vi "Chart[Template].Export.vi"(8 "error in (no error)":errorcluster, 10 "Export Folder Path":path, 11 "DisplayWaveforms":refnum<class "DisplayWaveforms.lvclass">) -> (0 "error out":errorcluster, 3 "DisplayWaveforms out":refnum<class "DisplayWaveforms.lvclass">)   [LabVIEW 2020, in "DisplayWaveform.lvlib" / "DisplayWaveforms.lvclass"]
doc: "Export Chart Data"
uses:
  DisplayWaveforms.lvclass
  DisplayWaveforms.lvclass/DisplayWaveforms.ctl
  <vilib>/Utility/file.llb/Write Delimited Spreadsheet (DBL).vi
panel:
  in  "Pause Charts":bool
  # "For instructions on how to use the JKI State Machine Objects, examples and video tutorials, visit:\nhttp://jki.net/state-machine-objects/\n\nJKI State Machine Objects™\nhttp://jki.net/state-machine-objects/\nCopyright (C) 2005-2015, JKI <info@jki.net>\nALL RIGHTS RESERVED"
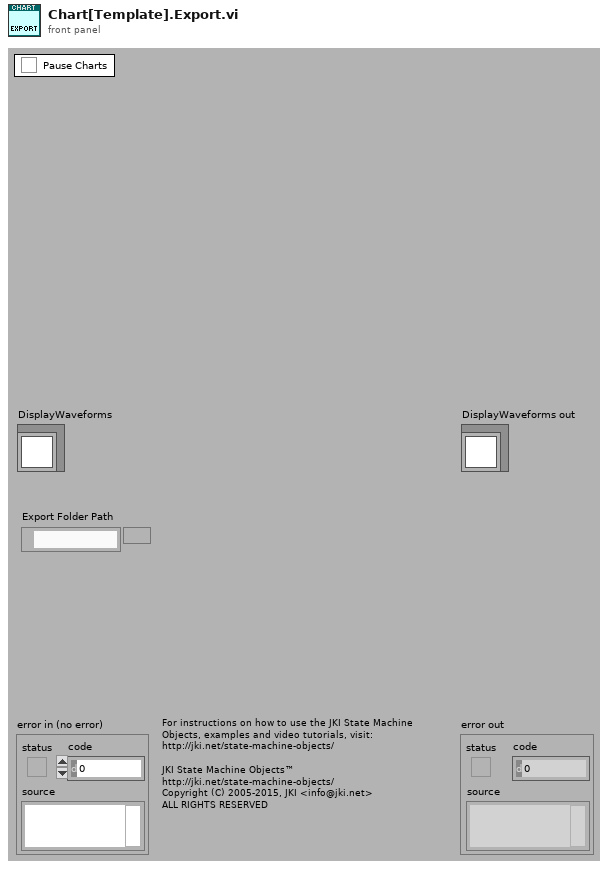
[diagram p1: front panel]
types:
  T1 = typedef "DisplayWaveform.lvlib/DisplayWaveforms.lvclass/PublicEvents--Cluster.ctl" = cluster{"Chart Cleared":refnum<user-event>, "Chart Exported":refnum<user-event>, "ChartParams Set":refnum<user-event>}
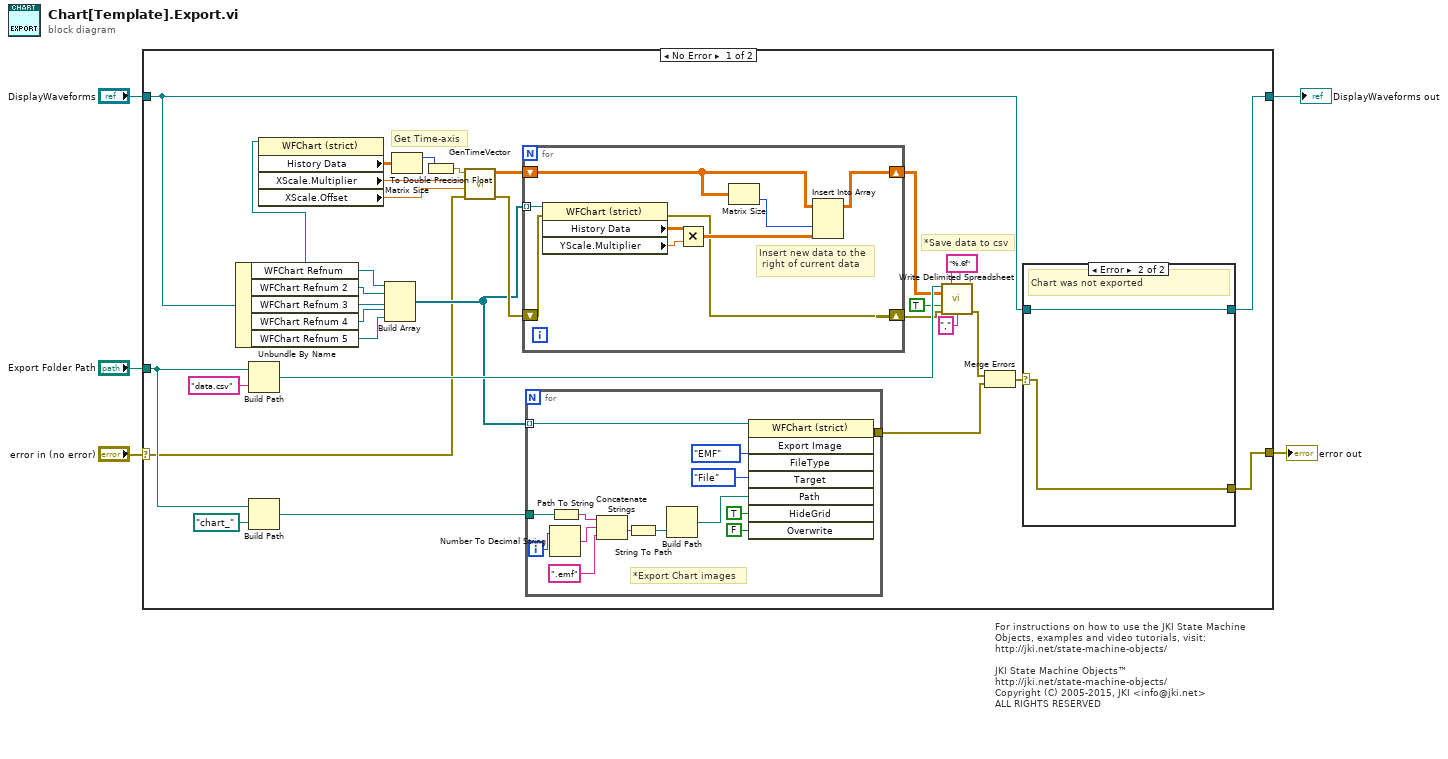
[diagram p0: block diagram]
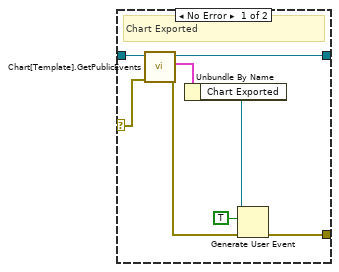
[diagram p2: hidden frame]
diagram:
  # "For instructions on how to use the JKI State Machine Objects, examples and video tutorials, visit:\nhttp://jki.net/state-machine-objects/\n\nJKI State Machine Objects™\nhttp://jki.net/state-machine-objects/\nCopyright (C) 2005-2015, JKI <info@jki.net>\nALL RIGHTS RESERVED"
  n1 = case shown="No Error" "error in (no error)" {
    selector: "error in (no error)" -> [w8 w69]
    tunnel: "DisplayWaveforms" -> [w27 w70]
    tunnel: [w35 w69] -> w4
    tunnel: [w34 w70] -> w3
    tunnel: "Export Folder Path" -> [w25 _]
    frame No Error {
      # "Get Time-axis"
      # "*Save data to csv"
      n2 = Unbundle By Name(w27) -> ("WFChart Refnum"=w24:refnum<vi>, "WFChart Refnum 2"=w23:refnum<vi>, "WFChart Refnum 3"=w22:refnum<vi>, "WFChart Refnum 4"=w21:refnum<vi>, "WFChart Refnum 5"=w20:refnum<vi>)
      n3 = Build Path(base path=w25, name or relative path="data.csv" ("string")) -> (appended path=w31:path)
      n4 = Build Path(base path=w25, name or relative path=path "chart_") -> (appended path=w17:path)
      n5 = property on="Property Node" class="WFChart (strict)"(reference=w24) -> ("History Data"=w32:dbl[][], "XScale.Multiplier"=w16:dbl, "XScale.Offset"=w15:dbl)  [unwired: 1 in, 2 out]
      n6 = Build Array(w24, w23, w22, w21, w20) -> (w9:refnum<vi>[])
      n7 = Matrix Size(0:w32) -> (1:w6:i32)  [unwired: 1 out]
      n8 = To Double Precision Float(number=w6) -> (double precision float=w14:dbl)
      n9 = call "GenTimeVector.vi"("error in (no error)"=w8, "Offset"=w15, "Multiplier - dT"=w16, "# of elements"=w14) -> ("error out"=w12:errorcluster, "Time Vector"=w13:dbl[][])  [unwired: 6 in]
      n10 = for {
        shift-right: [w39] -> w11
        shift-left: w13 -> [w42]
        shift-right: [w37] -> w10
        shift-left: w12 -> [w38]
        tunnel: w9 -> [w36] mode=indexing
        # "Insert new data to the\n right of current data"
        n11 = property on="Property Node" class="WFChart (strict)"(reference=w36, error in=w38) -> (error out=w37:errorcluster, "History Data"=w44:dbl[][], "YScale.Multiplier"=w43:dbl)  [unwired: 1 out]
        n12 = Multiply(x=w44, y=w43) -> (x*y=w40:dbl[][])
        n13 = Matrix Size(0:w42) -> (2:w41:i32)  [unwired: 1 out]
        n14 = Insert Into Array(array=w42, index (col)=w41, new element=w40) -> (w39:dbl[][])  [unwired: 1 in]
      }
      n15 = for {
        tunnel: w9 -> [w55] mode=indexing
        tunnel: [w54] -> w19
        tunnel: w17 -> [w46]
        i -> [w50]
        # "*Export Chart images"
        n16 = Number To Decimal String(number=w50) -> (decimal integer string=w49:string)  [unwired: 1 in]
        n17 = Path To String(path=w46) -> (string=w45:string)
        n18 = Concatenate Strings(w45, w49, ".emf" ("string")) -> (w51:string)
        n19 = String To Path(string=w51) -> (path=w52:path)
        n20 = Build Path(name or relative path=w52) -> (appended path=w47:path)  [unwired: 1 in]
        n21 = invoke on="Invoke Node" class="WFChart (strict)" method="Export Image"(reference=w55, "FileType"=enum32{"BMP", "EPS", "EMF", "PICT"}."EMF" ("File Type"), "Target"=enum32{"File", "Clipboard"}."File", "Path"=w47, "HideGrid"=TRUE ("Hide Grid"), "Overwrite"=FALSE ("Always Overwrite")) -> (error out=w54:errorcluster)  [unwired: 2 in, 7 out]
      }
      n22 = call-poly <vilib>:"Write Delimited Spreadsheet.vi"("file path (dialog if empty)"=w31, "format (%.3f)"="%.6f", "2D data"=w11, "append to file? (new file:F)"=TRUE, "error in (no error)"=w10, "delimiter (\\t)"="," ("delimiter (\\t)")) -> ("error out"=w29:errorcluster)  [unwired: 8 in, 1 out]
      n23 = Merge Errors(w29, w19) -> (w26:errorcluster)
      n24 = case shown="Error" w26 {
        selector: w26 -> [w59 w67]
        tunnel: [w62 w67] -> w35
        tunnel: w27 -> [w66 w68]
        tunnel: [w65 w68] -> w34
        frame No Error {
          # "Chart Exported"
          n25 = call "Chart[Template].GetPublicEvents.vi"("error in (no error)"=w59, "DisplayWaveforms"=w66) -> ("error out"=w63:errorcluster, "Chart[Template] Public Events"=w64:T1, "DisplayWaveforms out"=w65:refnum<class "DisplayWaveforms.lvclass">)  [unwired: 7 in]
          n26 = Unbundle By Name(w64) -> ("Chart Exported"=w60:refnum<user-event>)
          n27 = Generate User Event(user event=w60, event data cluster=TRUE ("event data"), error in=w63) -> (error out=w62:errorcluster)  [unwired: 1 in, 1 out]
        }
        frame Error {
          # "Chart was not exported"
        }
      }
    }
    frame Error {
    }
  }
  "error out" <- w4
  "DisplayWaveforms out" <- w3
